vi "acquire single wave by LAN subvi.vi"(4 "ID Query":string, 5 "Array 4":string[](array[string]), 6 "Array in":string[](array[string]), 7 "Array 3":string[](array[string]), 8 "error in (no error)":errorcluster, 9 "data in":string, 10 "Numeric":i32, 11 "TCP Network Connection in":refnum<k5>) -> (0 "Array out":i32[](array[numeric]), 1 "VOLTS/DIV":string, 2 "probe":string, 3 "scale":string)   [LabVIEW 2013]
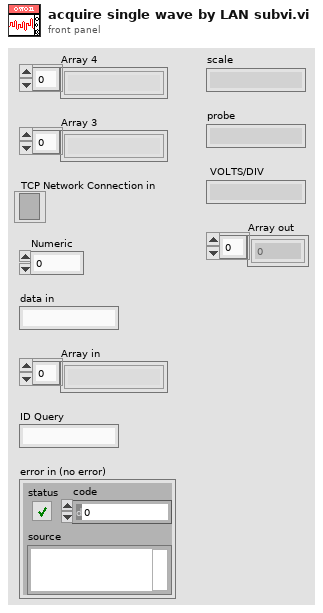
[diagram p1: front panel]
types:
  T1 = enum16{"Standard", "Buffered", "CRLF", "Immediate"}
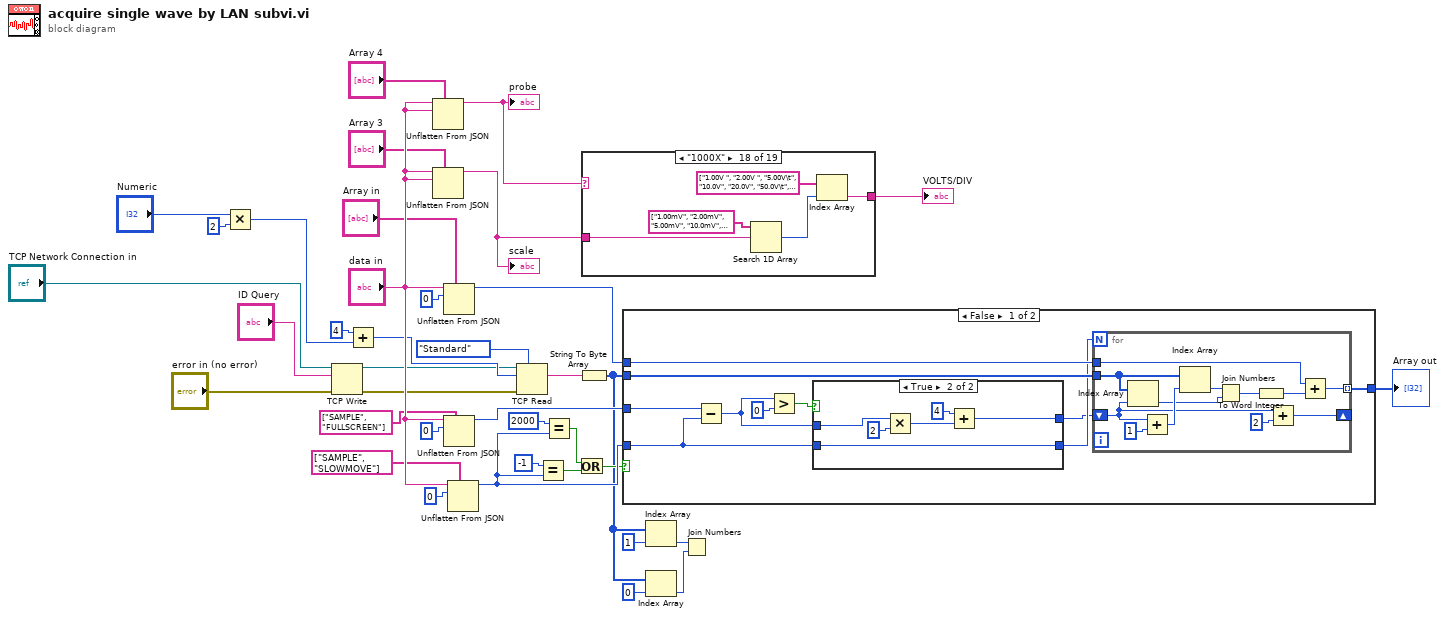
[diagram p0: block diagram]
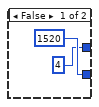
[diagram p2: hidden frame]
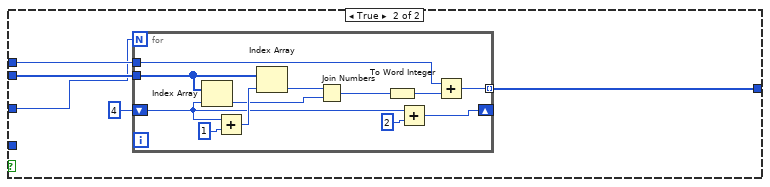
[diagram p3: hidden frame]
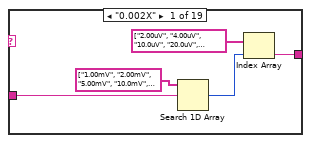
[diagram p4: hidden frame]
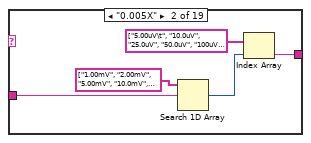
[diagram p5: hidden frame]
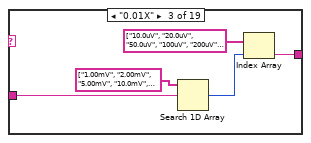
[diagram p6: hidden frame]
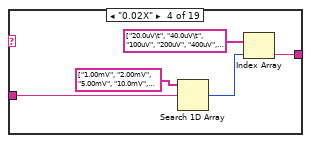
[diagram p7: hidden frame]
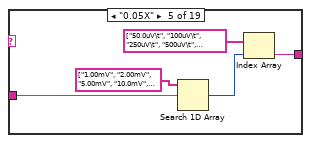
[diagram p8: hidden frame]
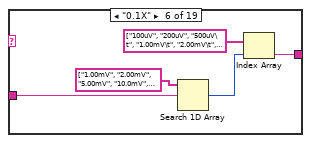
[diagram p9: hidden frame]
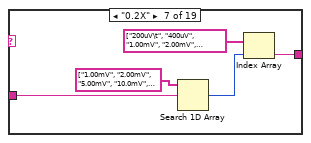
[diagram p10: hidden frame]
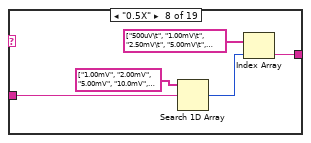
[diagram p11: hidden frame]
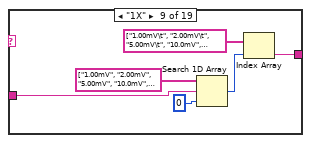
[diagram p12: hidden frame]
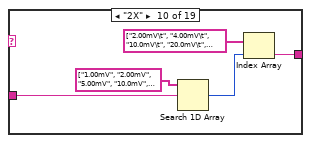
[diagram p13: hidden frame]
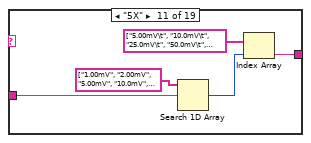
[diagram p14: hidden frame]
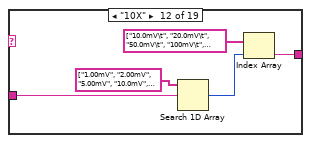
[diagram p15: hidden frame]
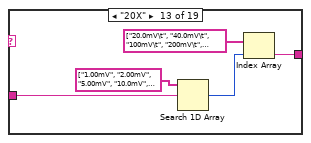
[diagram p16: hidden frame]
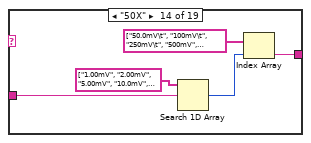
[diagram p17: hidden frame]
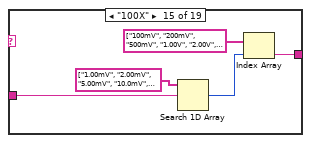
[diagram p18: hidden frame]
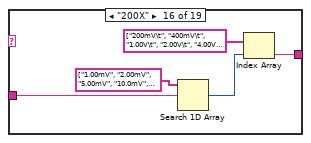
[diagram p19: hidden frame]
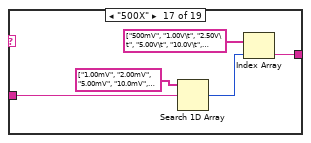
[diagram p20: hidden frame]
diagram:
  n1 = Multiply(x="Numeric", y=2) -> (x*y=w15:i32)
  n2 = TCP Write(connection ID="TCP Network Connection in", data in="ID Query", error in (no error)="error in (no error)") -> (connection ID out=w18:refnum<k5>, error out=w19:errorcluster)  [unwired: 1 in, 1 out]
  n3 = Add(x=4, y=w15) -> (x+y=w20:i32)
  n4 = Unflatten From JSON(path="Array 4", JSON string="data in", type and defaults="data in") -> (value=w23:string)  [unwired: 4 in, 1 out]
  "probe" <- w23
  n5 = Unflatten From JSON(path="Array 3", JSON string="data in", type and defaults="data in") -> (value=w24:string)  [unwired: 4 in, 1 out]
  "scale" <- w24
  n6 = Unflatten From JSON(path="Array in", JSON string="data in", type and defaults=0) -> (value=w12:i32)  [unwired: 4 in, 1 out]
  n7 = Unflatten From JSON(path=string[] ["SAMPLE", "FULLSCREEN"], JSON string="data in", type and defaults=0) -> (value=w34:i32)  [unwired: 4 in, 1 out]
  n8 = Unflatten From JSON(path=string[] ["SAMPLE", "SLOWMOVE"], JSON string="data in", type and defaults=0) -> (value=w37:i32)  [unwired: 4 in, 1 out]
  n9 = TCP Read(connection ID=w18, bytes to read=w20, error in (no error)=w19, 7:T1."Standard" ("mode (standard)")) -> (data out=w21:string)  [unwired: 1 in, 2 out]
  n10 = Equal?(x=-1, y=w37) -> (x = y?=w28:bool)
  n11 = Equal?(x=2000, y=w37) -> (x = y?=w27:bool)
  n12 = Or(x=w27, y=w28) -> (x .or. y?=w35:bool)
  n13 = String To Byte Array(string=w21) -> (unsigned byte array=w9:u8[])
  n14 = case shown="\"1000X\"" w23 {
    tunnel: w24 -> [w42 w47 w52 w57 w62 w67 w72 w77 w82 w88 w93 w98 w103 w108 w113 w118 w123 w128 w134]
    tunnel: [w41 w46 w51 w56 w61 w66 w71 w76 w81 w87 w92 w97 w102 w107 w112 w117 w122 w127 w131] -> w25
    frame "0.002X" {
      n15 = Search 1D Array(1D array=string[] ["1.00mV", "2.00mV", "5.00mV", "10.0mV", "20.0mV", "50.0mV", "100mV", "200mV", "500mV", "1.00V", "2.00V", "5.00V", "10.0V", "20.0V"], element=w42) -> (index of element=w43:i32)  [unwired: 1 in]
      n16 = Index Array(array=string[] ["2.00uV", "4.00uV", "10.0uV", "20.0uV", "50.0uV", "100uV", "200uV", "400uV", "1.00mV", "2.00mV\t", "4.00mV", "10.0mV", "20.0mV", "40.0mV"], index=w43) -> (element=w41:string)
    }
    frame "0.005X" {
      n17 = Search 1D Array(1D array=string[] ["1.00mV", "2.00mV", "5.00mV", "10.0mV", "20.0mV", "50.0mV", "100mV", "200mV", "500mV", "1.00V", "2.00V", "5.00V", "10.0V", "20.0V"], element=w47) -> (index of element=w48:i32)  [unwired: 1 in]
      n18 = Index Array(array=string[] ["5.00uV\t", "10.0uV", "25.0uV", "50.0uV", "100uV", "250uV", "500uV", "1.00mV\t", "2.50mV", "5.00mV", "10.0mV", "25.0mV", "50.0mV", "100mV"], index=w48) -> (element=w46:string)
    }
    frame "0.01X" {
      n19 = Search 1D Array(1D array=string[] ["1.00mV", "2.00mV", "5.00mV", "10.0mV", "20.0mV", "50.0mV", "100mV", "200mV", "500mV", "1.00V", "2.00V", "5.00V", "10.0V", "20.0V"], element=w52) -> (index of element=w53:i32)  [unwired: 1 in]
      n20 = Index Array(array=string[] ["10.0uV", "20.0uV", "50.0uV", "100uV", "200uV", "500uV", "1.00mV\t", "2.00mV\t", "5.00mV", "10.0mV\t", "20.0mV\t", "50.0mV", "100mV", "200mV"], index=w53) -> (element=w51:string)
    }
    frame "0.02X" {
      n21 = Search 1D Array(1D array=string[] ["1.00mV", "2.00mV", "5.00mV", "10.0mV", "20.0mV", "50.0mV", "100mV", "200mV", "500mV", "1.00V", "2.00V", "5.00V", "10.0V", "20.0V"], element=w57) -> (index of element=w58:i32)  [unwired: 1 in]
      n22 = Index Array(array=string[] ["20.0uV\t", "40.0uV\t", "100uV", "200uV", "400uV", "1.00mV", "2.00mV", "4.00mV", "10.0mV", "20.0mV", "40.0mV", "100mV", "200mV", "400mV"], index=w58) -> (element=w56:string)
    }
    frame "0.05X" {
      n23 = Search 1D Array(1D array=string[] ["1.00mV", "2.00mV", "5.00mV", "10.0mV", "20.0mV", "50.0mV", "100mV", "200mV", "500mV", "1.00V", "2.00V", "5.00V", "10.0V", "20.0V"], element=w62) -> (index of element=w63:i32)  [unwired: 1 in]
      n24 = Index Array(array=string[] ["50.0uV\t", "100uV\t", "250uV\t", "500uV\t", "1.00mV", "2.50mV\t", "5.00mV\t", "10.0mV\t", "25.0mV", "50.0mV\t", "100mV", "250mV", "500mV", "1.00V"], index=w63) -> (element=w61:string)
    }
    frame "0.1X" {
      n25 = Search 1D Array(1D array=string[] ["1.00mV", "2.00mV", "5.00mV", "10.0mV", "20.0mV", "50.0mV", "100mV", "200mV", "500mV", "1.00V", "2.00V", "5.00V", "10.0V", "20.0V"], element=w67) -> (index of element=w68:i32)  [unwired: 1 in]
      n26 = Index Array(array=string[] ["100uV", "200uV", "500uV\t", "1.00mV\t", "2.00mV\t", "5.00mV\t", "10.0mV\t", "20.0mV\t", "50.0mV\t", "100mV", "200mV", "500mV\t", "1.00V", "2.00V"], index=w68) -> (element=w66:string)
    }
    frame "0.2X" {
      n27 = Search 1D Array(1D array=string[] ["1.00mV", "2.00mV", "5.00mV", "10.0mV", "20.0mV", "50.0mV", "100mV", "200mV", "500mV", "1.00V", "2.00V", "5.00V", "10.0V", "20.0V"], element=w72) -> (index of element=w73:i32)  [unwired: 1 in]
      n28 = Index Array(array=string[] ["200uV\t", "400uV", "1.00mV", "2.00mV", "4.00mV\t", "10.0mV", "20.0mV", "40.0mV\t", "100mV", "200mV", "400mV", "1.00V", "2.00V", "4.00V"], index=w73) -> (element=w71:string)
    }
    frame "0.5X" {
      n29 = Search 1D Array(1D array=string[] ["1.00mV", "2.00mV", "5.00mV", "10.0mV", "20.0mV", "50.0mV", "100mV", "200mV", "500mV", "1.00V", "2.00V", "5.00V", "10.0V", "20.0V"], element=w77) -> (index of element=w78:i32)  [unwired: 1 in]
      n30 = Index Array(array=string[] ["500uV\t", "1.00mV\t", "2.50mV\t", "5.00mV\t", "10.0mV\t", "25.0mV\t", "50.0mV\t", "100mV", "250mV\t", "500mV\t", "1.00V\t", "2.50V\t", "5.00V\t", "10.0V"], index=w78) -> (element=w76:string)
    }
    frame "1X" {
      n31 = Search 1D Array(1D array=string[] ["1.00mV", "2.00mV", "5.00mV", "10.0mV", "20.0mV", "50.0mV", "100mV", "200mV", "500mV", "1.00V", "2.00V", "5.00V", "10.0V", "20.0V"], element=w82, start index (0)=0 ("开始索引(0)")) -> (index of element=w83:i32)
      n32 = Index Array(array=string[] ["1.00mV\t", "2.00mV\t", "5.00mV\t", "10.0mV", "20.0mV", "50.0mV", "100mV", "200mV\t", "500mV", "1.00V\t", "2.00V", "5.00V", "10.0V", "20.0V"], index=w83) -> (element=w81:string)
    }
    frame "2X" {
      n33 = Search 1D Array(1D array=string[] ["1.00mV", "2.00mV", "5.00mV", "10.0mV", "20.0mV", "50.0mV", "100mV", "200mV", "500mV", "1.00V", "2.00V", "5.00V", "10.0V", "20.0V"], element=w88) -> (index of element=w89:i32)  [unwired: 1 in]
      n34 = Index Array(array=string[] ["2.00mV\t", "4.00mV\t", "10.0mV\t", "20.0mV\t", "40.0mV", "100mV\t", "200mV", "400mV", "1.00V\t", "2.00V", "4.00V", "10.0V", "20.0V", "40.0V"], index=w89) -> (element=w87:string)
    }
    frame "5X" {
      n35 = Search 1D Array(1D array=string[] ["1.00mV", "2.00mV", "5.00mV", "10.0mV", "20.0mV", "50.0mV", "100mV", "200mV", "500mV", "1.00V", "2.00V", "5.00V", "10.0V", "20.0V"], element=w93) -> (index of element=w94:i32)  [unwired: 1 in]
      n36 = Index Array(array=string[] ["5.00mV\t", "10.0mV\t", "25.0mV\t", "50.0mV\t", "100mV\t", "250mV\t", "500mV", "1.00V", "2.50V\t", "5.00V", "10.0V\t", "25.0V", "50.0V ", "100V"], index=w94) -> (element=w92:string)
    }
    frame "10X" {
      n37 = Search 1D Array(1D array=string[] ["1.00mV", "2.00mV", "5.00mV", "10.0mV", "20.0mV", "50.0mV", "100mV", "200mV", "500mV", "1.00V", "2.00V", "5.00V", "10.0V", "20.0V"], element=w98) -> (index of element=w99:i32)  [unwired: 1 in]
      n38 = Index Array(array=string[] ["10.0mV\t", "20.0mV\t", "50.0mV\t", "100mV\t", "200mV", "500mV\t", "1.00V", "2.00V\t", "5.00V\t", "10.0V\t", "20.0V\t", "50.0V", "100V ", "200V"], index=w99) -> (element=w97:string)
    }
    frame "20X" {
      n39 = Search 1D Array(1D array=string[] ["1.00mV", "2.00mV", "5.00mV", "10.0mV", "20.0mV", "50.0mV", "100mV", "200mV", "500mV", "1.00V", "2.00V", "5.00V", "10.0V", "20.0V"], element=w103) -> (index of element=w104:i32)  [unwired: 1 in]
      n40 = Index Array(array=string[] ["20.0mV\t", "40.0mV\t", "100mV\t", "200mV\t", "400mV", "1.00V\t", "2.00V\t", "4.00V\t", "10.0V\t", "20.0V\t", "40.0V", "100V", "200V\t", "400V"], index=w104) -> (element=w102:string)
    }
    frame "50X" {
      n41 = Search 1D Array(1D array=string[] ["1.00mV", "2.00mV", "5.00mV", "10.0mV", "20.0mV", "50.0mV", "100mV", "200mV", "500mV", "1.00V", "2.00V", "5.00V", "10.0V", "20.0V"], element=w108) -> (index of element=w109:i32)  [unwired: 1 in]
      n42 = Index Array(array=string[] ["50.0mV\t", "100mV\t", "250mV\t", "500mV", "1.00V", "2.50V\t", "5.00V\t", "10.0V\t", "25.0V\t", "50.0V\t", "100V", "250V", "500V\t", "1.00kV"], index=w109) -> (element=w107:string)
    }
    frame "100X" {
      n43 = Search 1D Array(1D array=string[] ["1.00mV", "2.00mV", "5.00mV", "10.0mV", "20.0mV", "50.0mV", "100mV", "200mV", "500mV", "1.00V", "2.00V", "5.00V", "10.0V", "20.0V"], element=w113) -> (index of element=w114:i32)  [unwired: 1 in]
      n44 = Index Array(array=string[] ["100mV", "200mV", "500mV", "1.00V", "2.00V", "5.00V", "10.0V", "20.0V", "50.0V", "100V   ", "200V", "500V", "1.00kV\t", "2.00kV"], index=w114) -> (element=w112:string)
    }
    frame "200X" {
      n45 = Search 1D Array(1D array=string[] ["1.00mV", "2.00mV", "5.00mV", "10.0mV", "20.0mV", "50.0mV", "100mV", "200mV", "500mV", "1.00V", "2.00V", "5.00V", "10.0V", "20.0V"], element=w118) -> (index of element=w119:i32)  [unwired: 1 in]
      n46 = Index Array(array=string[] ["200mV\t", "400mV\t", "1.00V\t", "2.00V\t", "4.00V\t", "10.0V\t", "20.0V\t", "40.0V\t", "100V   ", "200V    ", "400V   ", "1.00kV", "2.00kV", "4.00kV"], index=w119) -> (element=w117:string)
    }
    frame "500X" {
      n47 = Search 1D Array(1D array=string[] ["1.00mV", "2.00mV", "5.00mV", "10.0mV", "20.0mV", "50.0mV", "100mV", "200mV", "500mV", "1.00V", "2.00V", "5.00V", "10.0V", "20.0V"], element=w123) -> (index of element=w124:i32)  [unwired: 1 in]
      n48 = Index Array(array=string[] ["500mV", "1.00V\t", "2.50V\t", "5.00V\t", "10.0V\t", "25.0V", "50.0V", "100V   ", "250V\t", "500V\t    ", "1.00kV\t", "2.50kV", "5.00kV", "10.0kV"], index=w124) -> (element=w122:string)
    }
    frame "1000X" {
      n49 = Search 1D Array(1D array=string[] ["1.00mV", "2.00mV", "5.00mV", "10.0mV", "20.0mV", "50.0mV", "100mV", "200mV", "500mV", "1.00V", "2.00V", "5.00V", "10.0V", "20.0V"], element=w128) -> (index of element=w129:i32)  [unwired: 1 in]
      n50 = Index Array(array=string[] ["1.00V ", "2.00V ", "5.00V\t", "10.0V", "20.0V", "50.0V\t", "100V", "200V  ", "500V   ", "1.00kV\t   ", "2.00kV ", "5.00kV\t", "10.0kV", "20.0kV"], index=w129) -> (element=w127:string)
    }
    frame "0.001X", Default {
      n51 = Search 1D Array(1D array=string[] ["1.00mV", "2.00mV", "5.00mV", "10.0mV", "20.0mV", "50.0mV", "100mV", "200mV", "500mV", "1.00V", "2.00V", "5.00V", "10.0V", "20.0V"], element=w134) -> (index of element=w133:i32)  [unwired: 1 in]
      n52 = Index Array(array=string[] ["1.00uV", "2.00uV", "5.00uV", "10.0uV", "20.0uV", "50.0uV,\t", "100uV,\t", "200uV,\t", "500uV,\t", "1.00mV,\t", "2.00mV,\t", "5.00mV,\t", "10.0mV, ", "20.0mv"], index=w133) -> (element=w131:string)
    }
  }
  "VOLTS/DIV" <- w25
  n53 = case shown="False" w35 {
    tunnel: w9 -> [w143 w169]
    tunnel: w12 -> [w142 w167]
    tunnel: [w144 w166] -> w38
    tunnel: w34 -> [w137 w165]
    tunnel: w37 -> [w138 _]
    frame False {
      n54 = Subtract(x=w137, y=w138) -> (x-y=w140:i32)
      n55 = Greater?(x=w140, y=0) -> (0:w139:bool)
      n56 = case shown="True" w139 {
        tunnel: [4 w151] -> w135
        tunnel: w140 -> [_ w148]
        tunnel: [1520 w147] -> w136
        tunnel: w138 -> [_ w147]
        frame False {
        }
        frame True {
          n57 = Multiply(x=w148, y=2) -> (x*y=w150:i32)
          n58 = Add(x=4, y=w150) -> (x+y=w151:i32)
        }
      }
      n59 = for {
        N: w136 -> [_]
        tunnel: w143 -> [w164]
        shift-right: [w161] -> _
        shift-left: w135 -> [w160]
        tunnel: [w158] -> w144 mode=indexing
        tunnel: w142 -> [w155]
        n60 = Index Array(array=w164, index=w160) -> (element=w156:u8)
        n61 = Add(x=w160, y=1) -> (x+y=w163:i32)
        n62 = Index Array(array=w164, index=w163) -> (element=w157:u8)
        n63 = Join Numbers(hi=w157, lo=w156) -> ((hi.lo)=w154:u16)
        n64 = To Word Integer(number=w154) -> (16bit integer=w153:i16)
        n65 = Add(x=w160, y=2) -> (x+y=w161:i32)
        n66 = Add(x=w155, y=w153) -> (x+y=w158:i32)
      }
    }
    frame True {
      n67 = for {
        N: w165 -> [_]
        tunnel: w169 -> [w181]
        shift-right: [w178] -> _
        shift-left: 4 -> [w177]
        tunnel: [w175] -> w166 mode=indexing
        tunnel: w167 -> [w172]
        n68 = Index Array(array=w181, index=w177) -> (element=w173:u8)
        n69 = Add(x=w177, y=1) -> (x+y=w180:i32)
        n70 = Index Array(array=w181, index=w180) -> (element=w174:u8)
        n71 = Join Numbers(hi=w174, lo=w173) -> ((hi.lo)=w171:u16)
        n72 = To Word Integer(number=w171) -> (16bit integer=w170:i16)
        n73 = Add(x=w177, y=2) -> (x+y=w178:i32)
        n74 = Add(x=w172, y=w170) -> (x+y=w175:i32)
      }
    }
  }
  "Array out" <- w38
  n75 = Index Array(array=w9, index=1) -> (element=w5:u8)
  n76 = Index Array(array=w9, index=0) -> (element=w6:u8)
  n77 = Join Numbers(hi=w5, lo=w6) -> ()  [unwired: 1 out]
